vi "ips120 switch heater.vi"(2 "wait interval (s)":dbl=10.0, 3 "error in (no error)":errorcluster, 4 "switch heater status":T1(ring), 5 "VISA resource name":refnum<visa-resource-name>) -> (0 "error out":errorcluster, 1 "VISA resource name 2":refnum<visa-resource-name>)   [LabVIEW 2013]
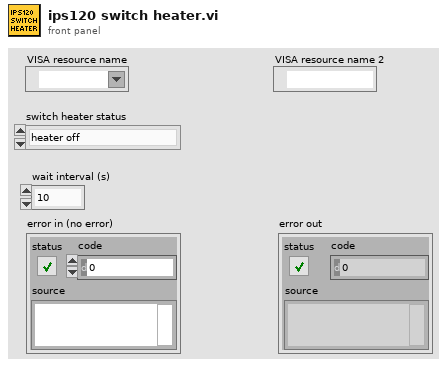
[diagram p1: front panel]
types:
  T1 = enum16{"heater off", "heater on psu=magnet", "heater on, no checks"}
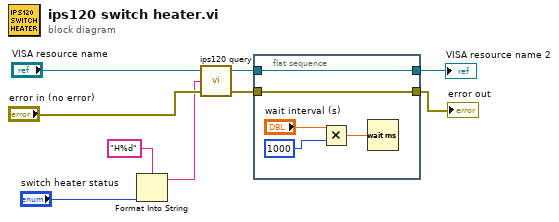
[diagram p0: block diagram]
diagram:
  n1 = Format Into String(format string="H%d", "switch heater status") -> (resulting string=w7:string)  [unwired: 2 in, 1 out]
  n2 = call "ips120 query.vi"("error in (no error)"="error in (no error)", "query"=w7, "VISA resource name"="VISA resource name") -> ("error out"=w2:errorcluster, "VISA resource name"=w4:refnum<visa-resource-name>)  [unwired: 1 out]
  n3 = flat-sequence {
    tunnel: w4 -> [w14]
    tunnel: [w14] -> w3
    tunnel: w2 -> [w13]
    tunnel: [w13] -> w1
    frame #0 {
      n4 = Multiply(x="wait interval (s)", y=1000) -> (x*y=w10:dbl)
      n5 = Wait (ms)(milliseconds to wait=w10) -> ()  [unwired: 1 out]
    }
  }
  "error out" <- w1
  "VISA resource name 2" <- w3
